vi "NI6071E.evt call Save DAQ Data.vi"(0 "i ref in":refnum<vi>, 2 "Client":string, 3 "Client timeout (10000)":i32=10000, 5 "error in (no error)":errorcluster) -> (14 "i ref out":refnum<vi>, 19 "error out":errorcluster)   [LabVIEW 2014, in "NI6071E.lvlib"]
doc: "This VI asks for an event by a simple call"
uses:
  NI6071E.lvlib
  CSCore/CSSystem/CoreLib/CoreLib.int 2 byte array.vi
  CSCore/BaseProcess/BaseProcess.lvlib
  CSCore/CSSystem/CoreLib/CoreLib.lvlib
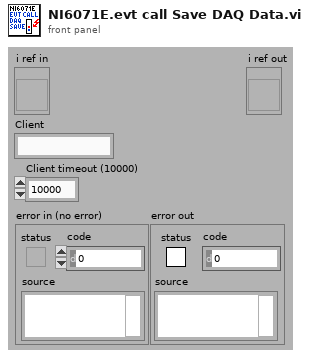
[diagram p1: front panel]
types:
  T1 = typedef "CoreDefs.rawDataType.ctl" = i8[]
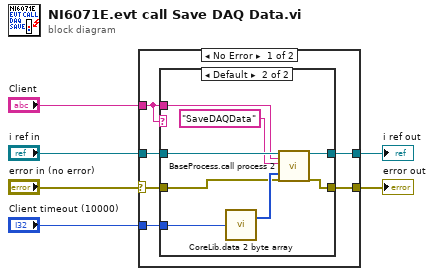
[diagram p0: block diagram]
diagram:
  n1 = case shown="No Error" "error in (no error)" {
    selector: "error in (no error)" -> [w7 w23]
    tunnel: "Client timeout (10000)" -> [w12 _]
    tunnel: [w11 w23] -> w5
    tunnel: "i ref in" -> [w10 w24]
    tunnel: "Client" -> [w8 _]
    tunnel: [w9 w24] -> w2
    frame No Error {
      n2 = case shown="Default" w8 {
        tunnel: w12 -> [_ w17]
        tunnel: w7 -> [w13 w15]
        tunnel: [w13 w22] -> w11
        tunnel: w10 -> [w14 w21]
        tunnel: w8 -> [_ w20]
        tunnel: [w14 w19] -> w9
        frame "N/A" {
        }
        frame Default {
          n3 = call-poly "CoreLib.data 2 byte array.vi"("i32"=w17) -> ("byteArray out"=w16:T1)  [unwired: 18 in]
          n4 = call "BaseProcess.call process 2.vi"("i ref in"=w21, "Object"=w20, "Selector"="SaveDAQData", "Data"=w16, "error in (no error)"=w15) -> ("i ref out"=w19:refnum<vi>, "error out"=w22:errorcluster)  [unwired: 13 in]
        }
      }
    }
    frame Error {
    }
  }
  "error out" <- w5
  "i ref out" <- w2
